vi "ArrayToFile.vi"(1 "Path Paramters":T2={"Parent Directory"=path "C:/", "Child Directory"=path "", "identifier"="", "name_base"="", "extension (\".psv\")"=".psv"}, 3 "Data cluster":cluster{"Data Array":dbl[], "2D-Array":dbl[][]}, 5 "Data Parameters":T1={"Array Type"=enum."2D", "delimiter (\"|\")"="|", "data format"="%.0f", "Filename Collision Handling"=enum."Increment"}, 6 "Save ?":bool=TRUE) -> (14 "target_filepath":path, 16 "Input Saved":bool, 18 "data_string":string)   [LabVIEW 2014]
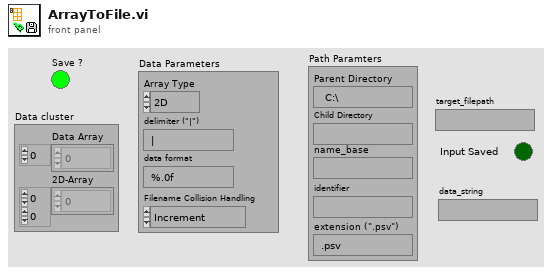
[diagram p1: front panel]
types:
  T1 = cluster{"Array Type":enum16{"2D", "row", "column"}, "delimiter (\"|\")":string, "data format":string, "Filename Collision Handling":enum16{"Increment", "Overwrite", "Treat as Error"}}
  T2 = cluster{"Parent Directory":path, "Child Directory":path, "identifier":string, "name_base":string, "extension (\".psv\")":string}
  T3 = enum16{"Increment", "Overwrite", "Treat as Error"}
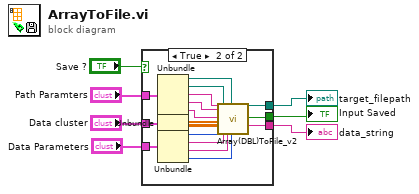
[diagram p0: block diagram]
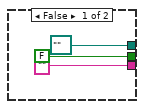
[diagram p2: hidden frame]
diagram:
  n1 = case shown="True" "Save ?" {
    tunnel: [FALSE ("Saved") w27] -> w7
    tunnel: ["" ("data_string") w26] -> w6
    tunnel: "Data Parameters" -> [_ w25]
    tunnel: "Data cluster" -> [_ w24]
    tunnel: "Path Paramters" -> [_ w23]
    tunnel: [path "" ("target_filepath") w11] -> w1
    frame False {
    }
    frame True {
      n2 = Unbundle(w23) -> ("Parent Directory"=w16:path, "Child Directory"=w17:path, "identifier"=w18:string, "name_base"=w19:string, "extension (\".psv\")"=w20:string)
      n3 = Unbundle(w24) -> ("Data Array"=w21:dbl[], "2D-Array"=w22:dbl[][])
      n4 = Unbundle(w25) -> ("Array Type"=w15:enum16{"2D", "row", "column"}, "delimiter (\"|\")"=w14:string, "data format"=w13:string, "Filename Collision Handling"=w12:T3)
      n5 = call "Array(DBL)ToFile_v2.vi"("name_base"=w18, "identifier(\"\")"=w19, "extension (\".psv\")"=w20, "1D-Array"=w21, "2D-Array"=w22, "Array Type (2D)"=w15, "Child Directory"=w17, "delimiter (\"|\")"=w14, "data format (DBL)"=w13, "Parent Directory"=w16, "Filename Collision Handling"=w12) -> ("target_filepath"=w11:path, "Saved"=w27:bool, "data_string"=w26:string)  [unwired: 14 in]
    }
  }
  "Input Saved" <- w7
  "data_string" <- w6
  "target_filepath" <- w1
